vi "telemetria.vi"(11 "Output Array":string[][](array[string])) -> (0 "v3":u16, 1 "sr v2":dbl format="%0.2f", 2 "v2":u16, 3 "œr v1":dbl format="%0.2f", 4 "sr v3":dbl format="%0.2f", 5 "v 1":u16, 6 "œrednie":T1, 8 "raw":cluster{u16, u16, u16, u16, u16, u16})   [LabVIEW 2014]
uses:
  <vilib>/ptbypt/NI_PtbyPt.lvlib
panel:
  out "resulting string":string
  out "string":string
  out "element 3":string
  out "œr v1  2":dbl format="%0.2f"
  out "sr v2 2":dbl format="%0.2f"
  out "v 2":u16
  out "v2 2":u16
  out "sr v3 2":dbl format="%0.2f"
  out "v3  2":u16
  out "element 2":string
  out "element":string
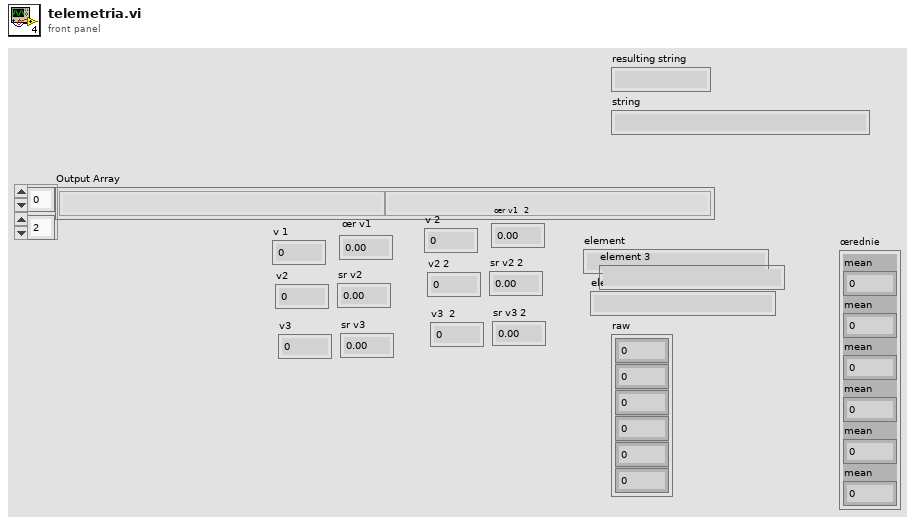
[diagram p1: front panel]
types:
  T1 = cluster{"mean":dbl, "mean":dbl, "mean":dbl, "mean":dbl, "mean":dbl, "mean":dbl}
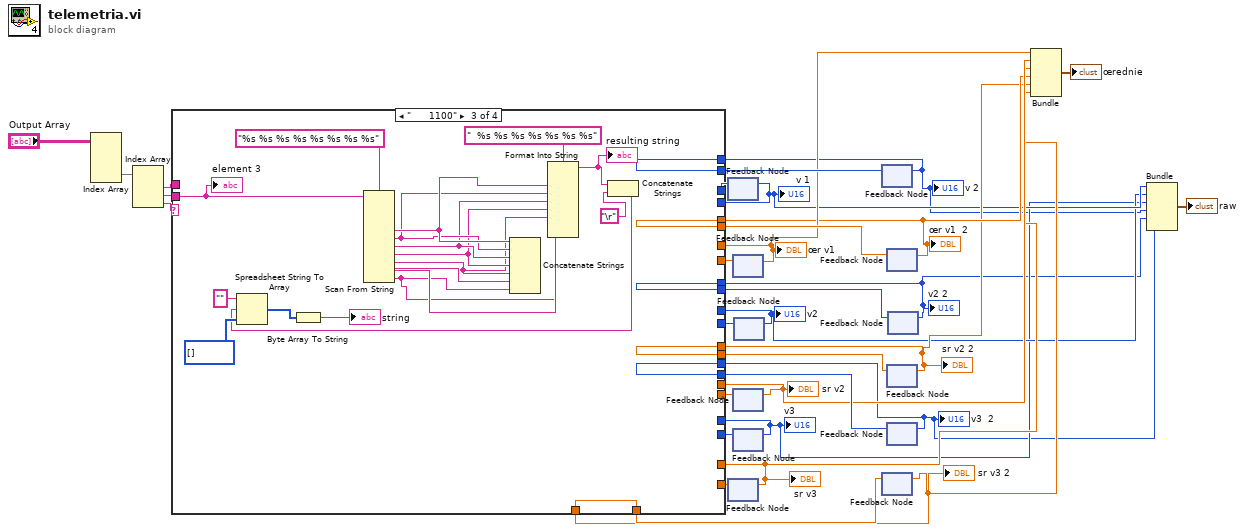
[diagram p0: block diagram]
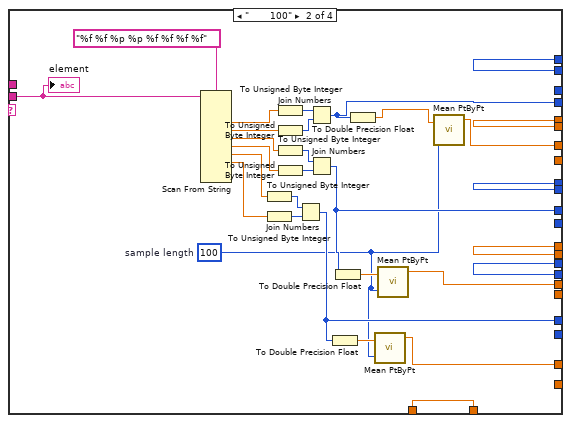
[diagram p3: hidden frame]
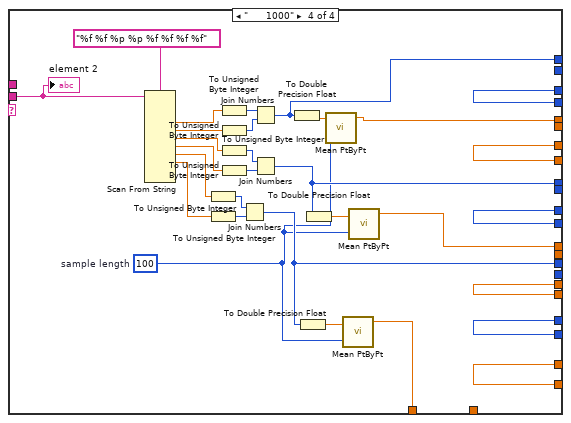
[diagram p4: hidden frame]
diagram:
  n1 = Index Array(array="Output Array") -> (element #2=w30:string[])  [unwired: 4 in, 1 out]
  n2 = Index Array(array=w30) -> (element #1=w23:string, element #2=w29:string, element #3=w28:string)  [unwired: 3 in]
  n3 = feedback #1() -> (w25:u16)  [unwired: 1 in]
  n4 = feedback #2() -> (w21:dbl)  [unwired: 1 in]
  n5 = feedback #3() -> (w26:dbl)  [unwired: 1 in]
  n6 = feedback #4() -> (w27:dbl)  [unwired: 1 in]
  n7 = feedback #5() -> (w22:u16)  [unwired: 1 in]
  n8 = feedback #6() -> (w24:u16)  [unwired: 1 in]
  n9 = feedback #7() -> (w20:u16)  [unwired: 1 in]
  n10 = feedback #8() -> (w15:dbl)  [unwired: 1 in]
  n11 = feedback #9() -> (w19:dbl)  [unwired: 1 in]
  n12 = feedback #10() -> (w17:dbl)  [unwired: 1 in]
  n13 = feedback #11() -> (w16:u16)  [unwired: 1 in]
  n14 = feedback #12() -> (w18:u16)  [unwired: 1 in]
  n15 = case shown="\"      1100\"" w28 {
    tunnel: w29 -> [_ w64 w89 w117]
    tunnel: [w42 w63 _ w102] -> w14
    tunnel: [w43 w62 _ w100] -> w13
    tunnel: w27 -> [w43 _ _ w100]
    tunnel: w26 -> [w42 _ _ w102]
    tunnel: [w41 w51 _ w103] -> w7
    tunnel: [w40 w61 _ w101] -> w6
    tunnel: w25 -> [w41 _ _ w103]
    tunnel: w24 -> [w40 _ _ w101]
    tunnel: w23 -> [_ _ _ _]
    tunnel: [w39 w54 _ w99] -> w5
    tunnel: [w38 w53 _ w98] -> w12
    tunnel: w22 -> [w39 _ _ w99]
    tunnel: w21 -> [w38 _ _ w98]
    tunnel: [w37 w50 w95 w109] -> w4
    tunnel: [w36 w49 w94 w108] -> w11
    tunnel: [w35 w48 w93 w107] -> w3
    tunnel: [w34 w47 w92 w106] -> w10
    tunnel: [w33 w46 w91 w105] -> w2
    tunnel: [w32 w45 w90 w104] -> w9
    tunnel: w20 -> [w37 w50 w95 _]
    tunnel: w19 -> [w36 w49 w94 _]
    tunnel: w18 -> [w35 w48 w93 _]
    tunnel: w17 -> [w34 w47 w92 _]
    tunnel: w16 -> [w33 w46 w91 _]
    tunnel: w15 -> [w32 w45 w90 _]
    frame "False", Default {
    }
    frame "       100" {
      w44 = 100  # sample length
      n16 = Scan From String(format string="%f %f %p %p %f %f %f %f", input string=w64) -> (output 1=w72:dbl, output 2=w71:dbl, output 3=w70:dbl, output 4=w67:dbl, output 5=w57:dbl, output 6=w56:dbl)  [unwired: 12 in, 3 out]
      n17 = To Unsigned Byte Integer(number=w57) -> (unsigned 8bit integer=w58:u8)
      n18 = To Unsigned Byte Integer(number=w56) -> (unsigned 8bit integer=w59:u8)
      n19 = To Unsigned Byte Integer(number=w72) -> (unsigned 8bit integer=w69:u8)
      n20 = To Unsigned Byte Integer(number=w71) -> (unsigned 8bit integer=w68:u8)
      n21 = To Unsigned Byte Integer(number=w70) -> (unsigned 8bit integer=w66:u8)
      n22 = To Unsigned Byte Integer(number=w67) -> (unsigned 8bit integer=w65:u8)
      n23 = Join Numbers(hi=w58, lo=w59) -> ((hi.lo)=w54:u16)
      n24 = Join Numbers(hi=w69, lo=w68) -> ((hi.lo)=w51:u16)
      n25 = Join Numbers(hi=w66, lo=w65) -> ((hi.lo)=w61:u16)
      n26 = To Double Precision Float(number=w54) -> (double precision float=w55:dbl)
      n27 = To Double Precision Float(number=w61) -> (double precision float=w60:dbl)
      n28 = To Double Precision Float(number=w51) -> (double precision float=w52:dbl)
      n29 = call <vilib>:"Mean PtByPt.vi"("x"=w55, "sample length"=w44) -> ("mean"=w53:dbl)  [unwired: 2 in, 1 out]
      n30 = call <vilib>:"Mean PtByPt.vi"("x"=w60, "sample length"=w44) -> ("mean"=w62:dbl)  [unwired: 2 in, 1 out]
      n31 = call <vilib>:"Mean PtByPt.vi"("x"=w52, "sample length"=w44) -> ("mean"=w63:dbl)  [unwired: 2 in, 1 out]
      "element" <- w64
    }
    frame "      1100" {
      n32 = Scan From String(format string="%s %s %s %s %s %s %s %s", input string=w89) -> (output 2=w84:string, output 3=w83:string, output 4=w82:string, output 5=w81:string, output 6=w80:string, output 7=w79:string, output 8=w78:string)  [unwired: 11 in, 3 out]
      n33 = Concatenate Strings(w84, w83, w82, w81, w80, w79, w78) -> ()  [unwired: 1 out]
      n34 = Format Into String(format string="  %s %s %s %s %s %s %s", w84, w83, w82, w81, w80, w79, w78) -> (resulting string=w76:string)  [unwired: 2 in, 1 out]
      "resulting string" <- w76
      n35 = Concatenate Strings(w76, "\r") -> (w74:string)
      n36 = Spreadsheet String To Array(format string="", spreadsheet string=w74, array type (2D Dbl)=u8[] [] ("unsigned byte array")) -> (array=w87:u8[])  [unwired: 1 in]
      n37 = Byte Array To String(unsigned byte array=w87) -> (string=→"string":string)
      "element 3" <- w89
    }
    frame "      1000" {
      w97 = 100  # sample length
      n38 = Scan From String(format string="%f %f %p %p %f %f %f %f", input string=w117) -> (output 1=w125:dbl, output 2=w124:dbl, output 3=w123:dbl, output 4=w120:dbl, output 5=w113:dbl, output 6=w112:dbl)  [unwired: 12 in, 3 out]
      n39 = To Unsigned Byte Integer(number=w113) -> (unsigned 8bit integer=w114:u8)
      n40 = To Unsigned Byte Integer(number=w112) -> (unsigned 8bit integer=w115:u8)
      n41 = To Unsigned Byte Integer(number=w125) -> (unsigned 8bit integer=w122:u8)
      n42 = To Unsigned Byte Integer(number=w124) -> (unsigned 8bit integer=w121:u8)
      n43 = To Unsigned Byte Integer(number=w123) -> (unsigned 8bit integer=w119:u8)
      n44 = To Unsigned Byte Integer(number=w120) -> (unsigned 8bit integer=w118:u8)
      n45 = Join Numbers(hi=w114, lo=w115) -> ((hi.lo)=w105:u16)
      n46 = Join Numbers(hi=w122, lo=w121) -> ((hi.lo)=w109:u16)
      n47 = Join Numbers(hi=w119, lo=w118) -> ((hi.lo)=w107:u16)
      n48 = To Double Precision Float(number=w109) -> (double precision float=w110:dbl)
      n49 = To Double Precision Float(number=w105) -> (double precision float=w111:dbl)
      n50 = To Double Precision Float(number=w107) -> (double precision float=w116:dbl)
      n51 = call <vilib>:"Mean PtByPt.vi"("x"=w110, "sample length"=w97) -> ("mean"=w108:dbl)  [unwired: 2 in, 1 out]
      n52 = call <vilib>:"Mean PtByPt.vi"("x"=w111, "sample length"=w97) -> ("mean"=w104:dbl)  [unwired: 2 in, 1 out]
      n53 = call <vilib>:"Mean PtByPt.vi"("x"=w116, "sample length"=w97) -> ("mean"=w106:dbl)  [unwired: 2 in, 1 out]
      "element 2" <- w117
    }
  }
  "œr v1" <- w14
  "sr v2" <- w13
  "v 1" <- w7
  "v2" <- w6
  "sr v3" <- w12
  "v3" <- w5
  "œr v1  2" <- w11
  "sr v2 2" <- w10
  "v 2" <- w4
  "v2 2" <- w3
  "sr v3 2" <- w9
  "v3  2" <- w2
  n54 = feedback-in #1(w7) -> ()
  n55 = feedback-in #2(w12) -> ()
  n56 = feedback-in #3(w14) -> ()
  n57 = feedback-in #4(w13) -> ()
  n58 = feedback-in #5(w5) -> ()
  n59 = feedback-in #6(w6) -> ()
  n60 = feedback-in #7(w4) -> ()
  n61 = feedback-in #8(w9) -> ()
  n62 = feedback-in #9(w11) -> ()
  n63 = feedback-in #10(w10) -> ()
  n64 = feedback-in #11(w2) -> ()
  n65 = feedback-in #12(w3) -> ()
  n66 = Bundle("mean"=w14, "mean"=w13, "mean"=w12, "mean"=w11, "mean"=w10, "mean"=w9) -> (→"œrednie":T1)  [unwired: 1 in]
  n67 = Bundle(w7, w6, w5, w4, w3, w2) -> (→"raw":cluster{u16, u16, u16, u16, u16, u16})  [unwired: 1 in]
